vi "upload_session.vi"(4 "chunk_size_bytes":i64=157286400, 6 "timeout_ms":i32=10000, 8 "error in (no error)":errorcluster, 9 "file":string, 10 "path":string, 11 "filepath":path) -> (0 "error out":errorcluster, 3 "filepath":string)   [LabVIEW 2015, in "lv-dropbox.lvlib" / "v2.lvlib"]
uses:
  v2.lvlib
  lv-dropbox.lvlib
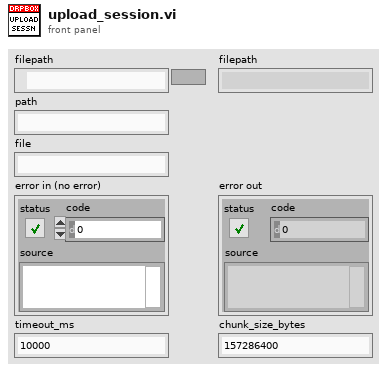
[diagram p1: front panel]
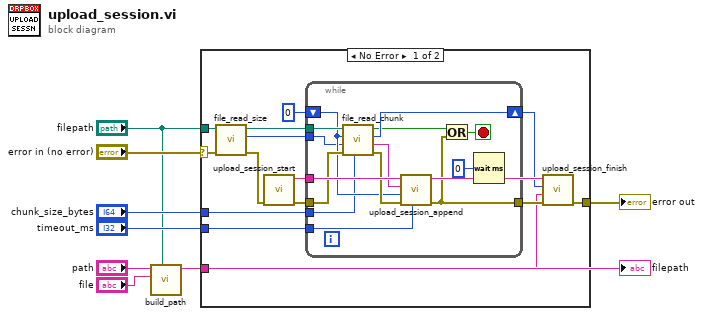
[diagram p0: block diagram]
diagram:
  n1 = call "build_path.vi"("filepath"="filepath", "path"="file", "base_path"="path") -> ("path"=w1:string)  [unwired: 8 in]
  "filepath" <- w1
  n2 = case shown="No Error" "error in (no error)" {
    selector: "error in (no error)" -> [w20 w36]
    tunnel: "filepath" -> [w10 _]
    tunnel: "timeout_ms" -> [w15 _]
    tunnel: [w12 w36] -> w6
    tunnel: "chunk_size_bytes" -> [w11 _]
    tunnel: w1 -> [w9 _]
    frame No Error {
      n3 = call "file_read_size.vi"("error in (no error)"=w20, "filepath"=w10) -> ("error out"=w21:errorcluster, "size_bytes"=w16:i64)  [unwired: 8 in]
      n4 = call "upload_session_start.vi"("error in (no error)"=w21) -> ("error out"=w17:errorcluster, "session_id"=w18:string)  [unwired: 9 in]
      n5 = while {
        shift-right: [w27] -> w13
        shift-left: i64 0 -> [w26]
        tunnel: w18 -> [w32]
        tunnel: w16 -> [w23]
        tunnel: w15 -> [w31]
        tunnel: w10 -> [w28]
        tunnel: w11 -> [w24]
        tunnel: w17 -> [w35]
        tunnel: [w30] -> w14
        stop <- w29 stop-if-true
        n6 = call "file_read_chunk.vi"("chunk_size_bytes"=w24, "error in (no error)"=w35, "file_size"=w23, "offset_in"=w26, "filepath"=w28) -> ("error out"=w34:errorcluster, "data"=w33:string, "offset_out"=w27:i64, "last_chunk"=w22:bool)  [unwired: 3 in]
        n7 = call "upload_session_append.vi"("timeout_ms"=w31, "error in (no error)"=w34, "offset"=w26, "data"=w33, "session_id"=w32) -> ("error out"=w30:errorcluster)  [unwired: 6 in]
        n8 = Or(x=w22, y=w30) -> (x .or. y?=w29:bool)
        n9 = Wait (ms)(milliseconds to wait=u32 0) -> ()  [unwired: 1 out]
      }
      n10 = call "upload_session_finish.vi"("error in (no error)"=w14, "path"=w9, "offset"=w13, "session_id"=w18) -> ("error out"=w12:errorcluster)  [unwired: 7 in]
    }
    frame Error {
    }
  }
  "error out" <- w6
